vi "Read Message.vi"(8 "error in (no error)":errorcluster, 11 "TraceMessage in":refnum<class "Trace.lvclass">) -> (0 "error out":errorcluster, 2 "Message":string, 3 "TraceMessage out":refnum<class "Trace.lvclass">)   [LabVIEW 2013, in "Trace.lvclass"]
uses:
  Trace.lvclass
  Trace.lvclass/Trace.ctl
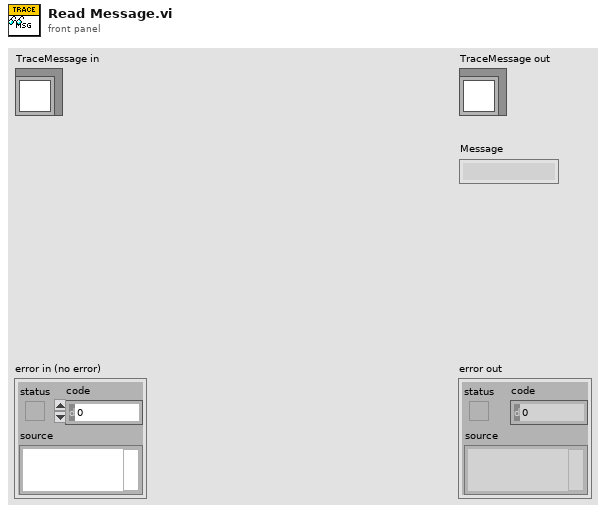
[diagram p1: front panel]
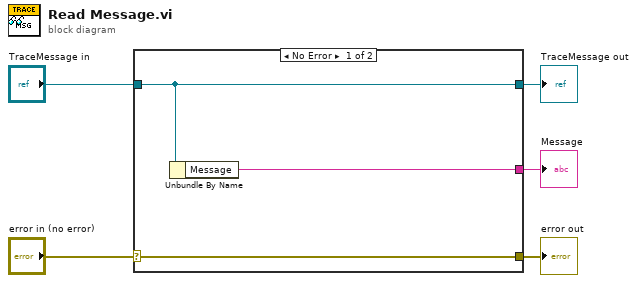
[diagram p0: block diagram]
diagram:
  n1 = case shown="No Error" "error in (no error)" {
    selector: "error in (no error)" -> [w8 w9]
    tunnel: [w8 w9] -> w4
    tunnel: [w7 w10] -> w2
    tunnel: "TraceMessage in" -> [w7 w10]
    tunnel: [w6 _] -> w1
    frame No Error {
      n2 = Unbundle By Name(w7) -> ("Message"=w6:string)
    }
    frame Error {
    }
  }
  "error out" <- w4
  "TraceMessage out" <- w2
  "Message" <- w1
